vi "TR_ManageVIActivation.vi"(11 "Menu in":refnum<class "VIActivation.lvclass">) -> ()   [LabVIEW 2021, in "VIActivation.lvlib" / "VIActivation.lvclass"]
uses:
  VIActivation.lvclass
  687d16a6-6148-407a-a2d8-39ae7b2e2ec5.vi
  VIActivationEvents.ctl
  ClassUtilities/src/ClassByRef/ClassByRef.lvclass
  <vilib>/ErrorRing/Error Ring.xnode
  C:/Users/Dany/OneDrive/LabVIEW/Class/ClassUtilities/ClassByRef/ClassByRef.lvclass
  C:/Users/Dany/OneDrive/LabVIEW/Class/VIActivation/VIActivation.lvclass
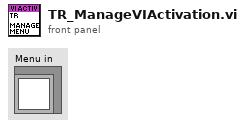
[diagram p1: front panel]
types:
  T1 = typedef "VIActivation.lvlib/VIActivation.lvclass/VIActivationEvents.ctl" = cluster{"AppRef":refnum<vi>, "VIName":string, "VIWindow":i32, "VIAppRef":refnum<vi>}
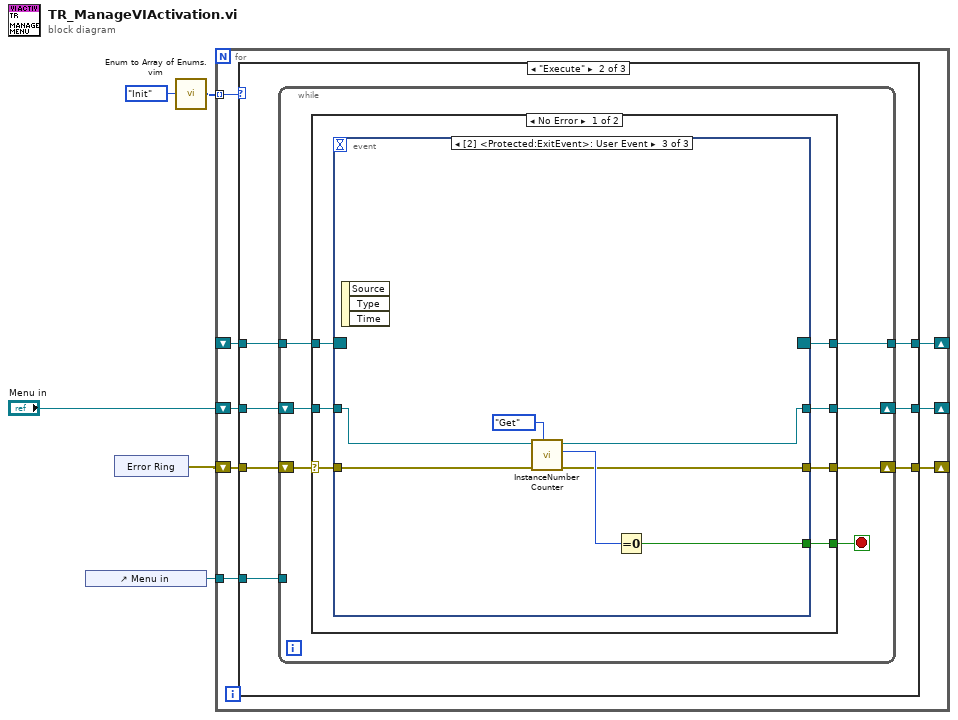
[diagram p0: block diagram]
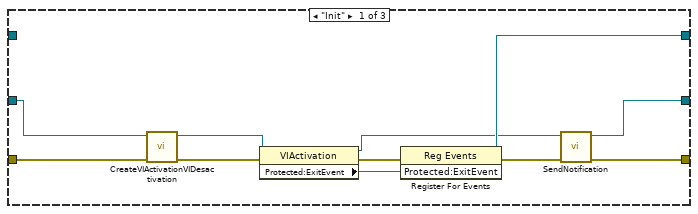
[diagram p2: hidden frame]
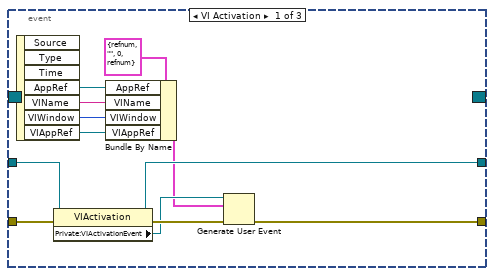
[diagram p3: hidden frame]
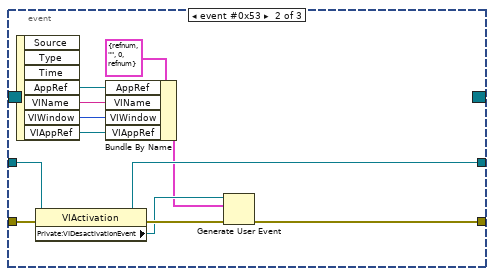
[diagram p4: hidden frame]
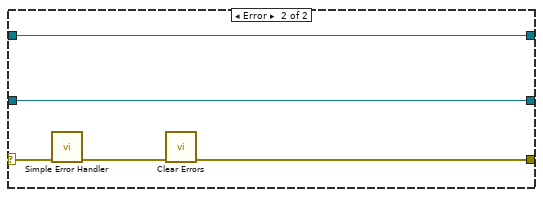
[diagram p5: hidden frame]
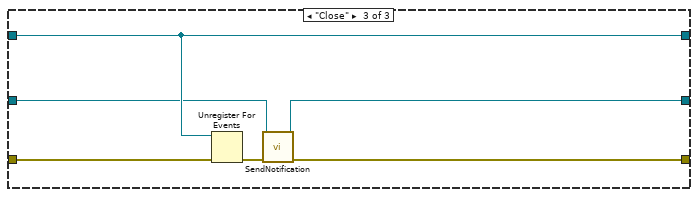
[diagram p6: hidden frame]
diagram:
  n1 = control-ref of="Menu in"() -> (w5:refnum<vi>)
  n2 = xnode "Error Ring"() -> ("error out"=w1:errorcluster)
  n3 = call "Enum to Array of Enums.vim"("enum"=enum16{"Init", "Execute", "Close"}."Init") -> ("array of enums"=w3:enum16{"Init", "Execute", "Close"}[])
  n4 = for {
    tunnel: w5 -> [w12]
    shift-right: [w10] -> _
    shift-left: w1 -> [w13]
    tunnel: w3 -> [w11] mode=indexing
    shift-right: [w8] -> _
    shift-left: "Menu in" -> [w9]
    shift-right: [w7] -> _
    shift-left: _ -> [w6]
    n5 = case shown="\"Execute\"" w11 {
      tunnel: w13 -> [w24 w31 w87]
      tunnel: [w19 w30 w84] -> w10
      tunnel: w12 -> [_ w29 _]
      tunnel: w9 -> [w23 w27 w82]
      tunnel: [w21 w28 w83] -> w8
      tunnel: [w22 w25 w85] -> w7
      tunnel: w6 -> [_ w26 w85]
      frame "Init" {
        n6 = call "CreateVIActivationVIDesactivation.vi"("error in (no error)"=w24, "Menu in"=w23) -> ("error out"=w18:errorcluster, "Menu out"=w17:refnum<class "VIActivation.lvclass">)  [unwired: 8 in]
        n7 = property class="VIActivation"(reference=w17, error in=w18) -> (reference out=w16:refnum<class "VIActivation.lvclass">, error out=w15:errorcluster, "Protected:ExitEvent"=w14:refnum<user-event>)
        n8 = register-events(error in=w15, w14) -> (reference out=w22:refnum<event-registration>, error out=w20:errorcluster)  [unwired: 1 in]
        n9 = call "SendNotification.vi"("error in (no error)"=w20, "ByRefClass in"=w16) -> ("error out"=w19:errorcluster, "ByRefClass out"=w21:refnum<class "VIActivation.lvclass">)  [unwired: 8 in]
      }
      frame "Execute" {
        n10 = while {
          shift-right: [w35] -> w28
          shift-left: w27 -> [w38]
          shift-right: [w36] -> w30
          shift-left: w31 -> [w37]
          tunnel: w29 -> [_]
          tunnel: w26 -> [w33]
          tunnel: [w32] -> w25
          stop <- w34 stop-if-true
          n11 = case shown="No Error" w37 {
            selector: w37 -> [w44 w81]
            tunnel: w38 -> [w45 w80]
            tunnel: [w43 w78] -> w36
            tunnel: [w42 w80] -> w35
            tunnel: [w41 _] -> w34
            tunnel: w33 -> [w39 w77]
            tunnel: [w40 w77] -> w32
            frame No Error {
              n12 = event shown="[2] <Protected:ExitEvent>: User Event" {
                selector: w39 -> [_ _ _]
                dyn-events: [_ _ _] -> w40
                timeout: _ -> [_ _ _]
                tunnel: w45 -> [w56 w68 w71]
                tunnel: w44 -> [w57 w69 w74]
                tunnel: [w53 w65 w73] -> w43
                tunnel: [w55 w67 w72] -> w42
                tunnel: [_ _ w70] -> w41
                event VI Activation {
                  n13 = event-data() -> ("AppRef"=w50:refnum<vi>, "VIName"=w49:string, "VIWindow"=w48:i32, "VIAppRef"=w47:refnum<vi>)  [unwired: 1 in, 3 out]
                  n14 = property class="VIActivation"(reference=w56, error in=w57) -> (reference out=w55:refnum<class "VIActivation.lvclass">, error out=w54:errorcluster, "Private:VIActivationEvent"=w52:refnum<user-event>)
                  n15 = Bundle By Name(cluster=T1 {"AppRef"=refnum, "VIName"="", "VIWindow"=0, "VIAppRef"=refnum} ("VI Activation"), "AppRef"=w50, "VIName"=w49, "VIWindow"=w48, "VIAppRef"=w47) -> (w51:T1)
                  n16 = Generate User Event(user event=w52, event data cluster=w51, error in=w54) -> (error out=w53:errorcluster)  [unwired: 1 in, 1 out]
                }
                event event #0x53 {
                  n17 = event-data() -> ("AppRef"=w62:refnum<vi>, "VIName"=w61:string, "VIWindow"=w60:i32, "VIAppRef"=w59:refnum<vi>)  [unwired: 1 in, 3 out]
                  n18 = property class="VIActivation"(reference=w68, error in=w69) -> (reference out=w67:refnum<class "VIActivation.lvclass">, error out=w66:errorcluster, "Private:VIDesactivationEvent"=w64:refnum<user-event>)
                  n19 = Bundle By Name(cluster=T1 {"AppRef"=refnum, "VIName"="", "VIWindow"=0, "VIAppRef"=refnum} ("VI Activation"), "AppRef"=w62, "VIName"=w61, "VIWindow"=w60, "VIAppRef"=w59) -> (w63:T1)
                  n20 = Generate User Event(user event=w64, event data cluster=w63, error in=w66) -> (error out=w65:errorcluster)  [unwired: 1 in, 1 out]
                }
                event User Event {
                  n21 = event-data() -> ()  [unwired: 1 in, 3 out]
                  n22 = call "InstanceNumberCounter.vi"("Action"=enum16{"Get", "Add", "Subtract"}."Get", "error in (no error)"=w74, "VI Activation in"=w71) -> ("error out"=w73:errorcluster, "InstanceNumber out"=w76:i32, "VI Activation out"=w72:refnum<class "VIActivation.lvclass">)  [unwired: 6 in]
                  n23 = Equal To 0?(x=w76) -> (x = 0?=w70:bool)
                }
              }
            }
            frame Error {
              n24 = call <vilib>:"Simple Error Handler.vi"("error in (no error)"=w81) -> ("error out"=w79:errorcluster)  [unwired: 4 in, 4 out]
              n25 = call <vilib>:"Clear Errors.vi"("error in (no error)"=w79) -> ("error out"=w78:errorcluster)  [unwired: 5 in, 1 out]
            }
          }
        }
      }
      frame "Close" {
        n26 = Unregister For Events(event registration refnum=w85, error in=w87) -> (error out=w86:errorcluster)
        n27 = call "SendNotification.vi"("error in (no error)"=w86, "ByRefClass in"=w82) -> ("error out"=w84:errorcluster, "ByRefClass out"=w83:refnum<class "VIActivation.lvclass">)  [unwired: 8 in]
      }
    }
  }
